vi "Get Version.vi"(11 "error in (no error)":errorcluster) -> (4 "Version information":string, 6 "Connected?":bool, 15 "error out":errorcluster)   [LabVIEW 2024, in "GRBL 1.1.lvlib"]
doc: "Show the GRBL version and source code build date."
uses:
  GRBL 1.1.lvlib
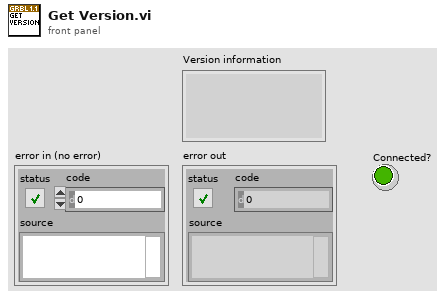
[diagram p1: front panel]
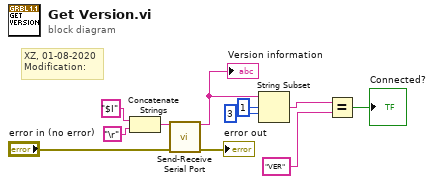
[diagram p0: block diagram]
diagram:
  # "XZ, 01-08-2020\nModification:"
  n1 = Concatenate Strings("$I" ("Data to write"), "\r") -> (w9:string)
  n2 = call "Send-Receive Serial Port.vi"("Data to write"=w9, "error in (no error)"="error in (no error)") -> ("Data read"=w4:string, "error out"=→"error out":errorcluster)  [unwired: 12 in]
  "Version information" <- w4
  n3 = String Subset(string=w4, offset (0)=1, length (rest)=3 ("length (rest)")) -> (substring=w3:string)
  n4 = Equal?(x=w3, y="VER" ("Version information")) -> (x = y?=→"Connected?":bool)
